vi "PromptForAttributes.vi"(9 "Attributes In":string[][](array[string]), 10 "Mouse Coords":T1, 11 "New Node Name":string) -> (2 "Canceled":bool, 3 "Attributes":string[][](array[string]))   [LabVIEW 2020]
uses:
  <vilib>/Utility/miscctls.llb/LVPoint32TypeDef.ctl
  Utils/FilePath.vi
  <vilib>/Utility/Data Type/NI_Data Type.lvlib
panel:
  out "Array":variant[](array[variant])
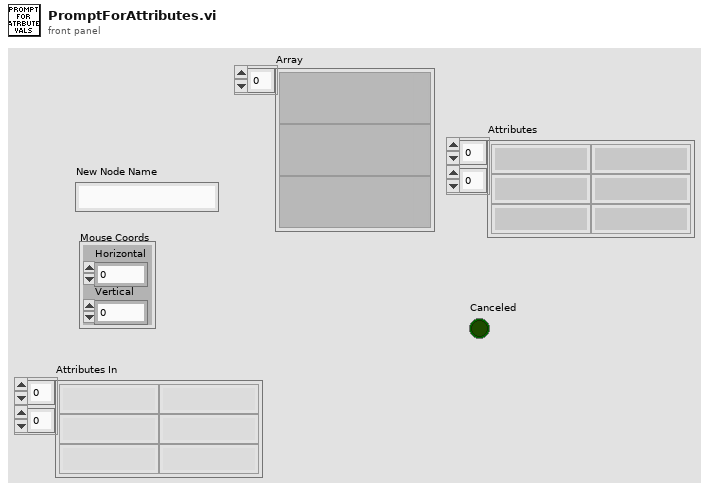
[diagram p1: front panel]
types:
  T1 = typedef "LVPoint32TypeDef.ctl" = cluster{"Horizontal":i32, "Vertical":i32}
  T2 = cluster{"Horizontal":i32, "Vertical":i32, "Horizontal":i32, "Vertical":i32}
  T3 = typedef "NI_Data Type.lvlib/Data Type.ctl" = enum8{"Invalid Type", "Void", "I8", "I16", "I32", "I64", "U8", "U16", "U32", "U64", "Single Float", "Double Float", "Extended Float", "Single Complex", "Double Complex", "Extended Complex", "Enum U8", "Enum U16", "Enum U32", "Enum U64", "Single Float With Unit", "Double Float With Unit", "Extended Float With Unit", "Single Complex with Unit", "Double Complex with Unit", "Extended Complex with Unit", "Boolean", "String", "Path", "Picture", "Tag", "Array", "Cluster", "Variant", "LV Variant", "Waveform", "Timestamp", "Digital Waveform", "Digital Data", "ExpressData", "Refnum", "External Data", "VI", "Poly VI", "LabVIEW Class Instance", "Fixed Point", "Set Collection", "Map Collection"}
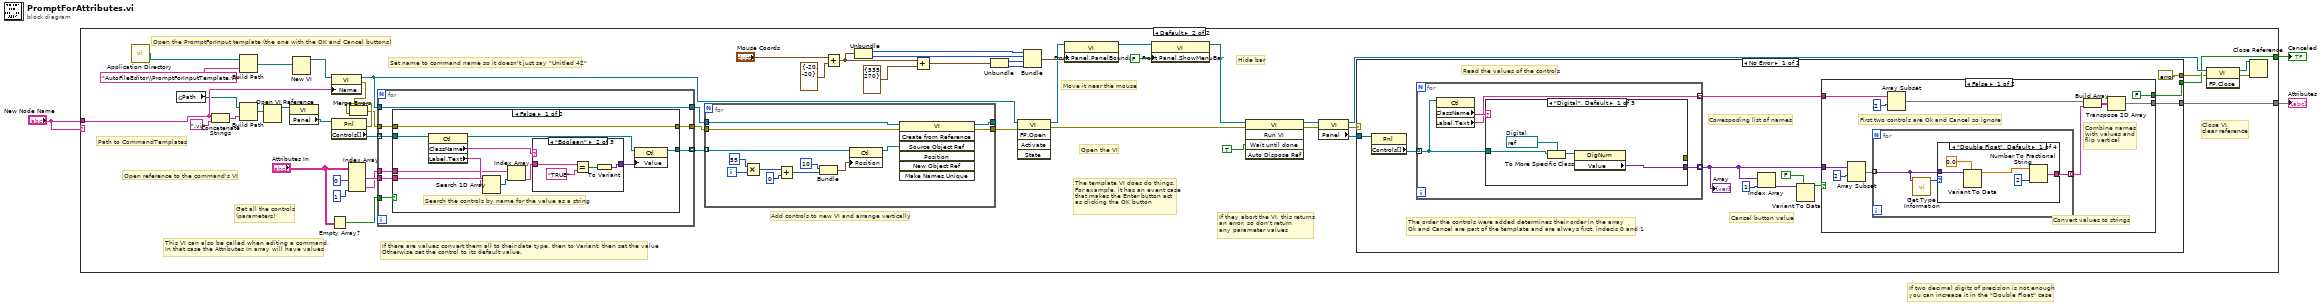
[diagram p0: block diagram]
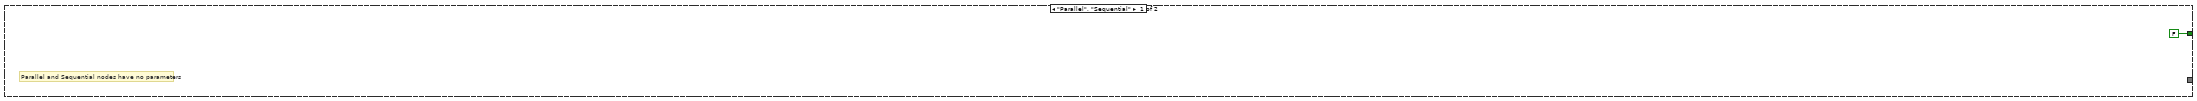
[diagram p2: hidden frame]
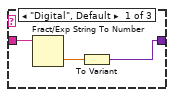
[diagram p3: hidden frame]
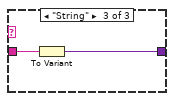
[diagram p4: hidden frame]
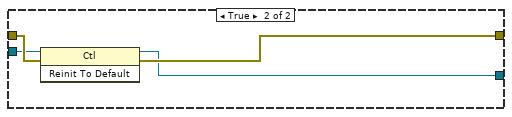
[diagram p5: hidden frame]
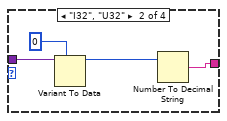
[diagram p6: hidden frame]
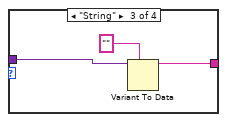
[diagram p7: hidden frame]
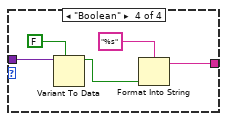
[diagram p8: hidden frame]
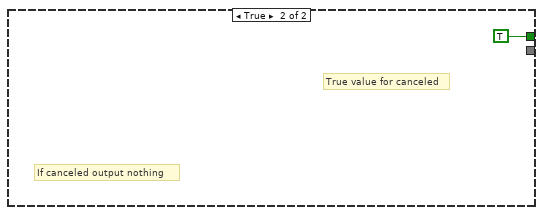
[diagram p9: hidden frame]
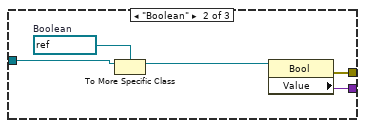
[diagram p10: hidden frame]
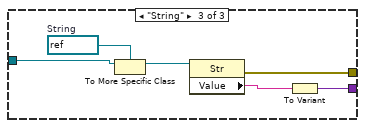
[diagram p11: hidden frame]
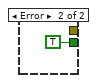
[diagram p12: hidden frame]
diagram:
  # "If two decimal digits of precision is not enough\nyou can increase it in the \"Double Float\" case"
  n1 = case shown="Default" "New Node Name" {
    tunnel: "New Node Name" -> [_ w13]
    tunnel: [FALSE ("Canceled") w42] -> w3
    tunnel: [_ w41] -> w2
    frame "Parallel", "Sequential" {
      # "Parallel and Sequential nodes have no parameters"
    }
    frame Default {
      # "The template VI does do things.\nFor example, it has an event case\nthat makes the Enter button act\nas clicking the OK button"
      # "Hide bar"
      # "Close VI,\nclear reference"
      # "If there are values convert them all to their data type, then to Variant, then set the value\nOtherwise set the control to its default value."
      # "This VI can also be called when editing a command.\nIn that case the Attributes In array will have values"
      # "Set name to command name so it doesn't just say \"Unitled 42\""
      # "Open the VI"
      # "Get all the controls\n(parameters)"
      # "Path to CommandTemplates"
      # "If they abort the VI, this returns\nan error, so don't return\nany parameter values"
      # "Open reference to the command's VI"
      # "Move it near the mouse"
      # "Add controls to new VI and arrange vertically"
      # "Open the PromptForInput template (the one with the OK and Cancel buttons)"
      n2 = call <vilib>:"Application Directory.vi"() -> ("Application Directory"=w11:path)
      n3 = global read "FilePath.vi" "Path"() -> (w12:path)
      n4 = Concatenate Strings(w13, ".vi" ("string")) -> (w45:string)
      n5 = Build Path(base path=w11, name or relative path="AutoFileEditor\\PromptForInputTemplate.vi") -> (appended path=w47:path)
      n6 = Build Path(base path=w12, name or relative path=w45) -> (appended path=w44:path)
      n7 = Open VI Reference(vi path=w44) -> (vi reference=w26:refnum<vi>)  [unwired: 5 in, 1 out]
      n8 = property class="VI"(reference=w26) -> ("Panel"=w56:refnum<vi>)  [unwired: 1 in, 2 out]
      n9 = New VI(10:w47) -> (3:w51:refnum<vi>)  [unwired: 6 in, 1 out]
      n10 = Empty Array?(array="Attributes In") -> (empty?=w14:bool)
      n11 = property class="Pnl"(reference=w56) -> (error out=w9:errorcluster, "Controls[]"=w22:refnum<vi>[])  [unwired: 1 in, 1 out]
      n12 = property class="VI"(reference=w51, "Name"=w13) -> (reference out=w5:refnum<vi>, error out=w8:errorcluster)  [unwired: 1 in]
      n13 = Index Array(array="Attributes In", index (col) #1=0 ("disabled index (col)"), index (col) #2=1 ("index (col)")) -> (element #1=w18:string[], element #2=w16:string[])  [unwired: 2 in]
      n14 = Merge Errors(w8, w9) -> (w7:errorcluster)
      n15 = for {
        tunnel: w22 -> [w62] mode=indexing
        tunnel: [w63] -> w21 mode=indexing
        tunnel: [w57] -> w20
        tunnel: w7 -> [w58]
        tunnel: [w64] -> w6
        tunnel: w5 -> [w64]
        tunnel: w18 -> [w61]
        tunnel: w16 -> [w60]
        tunnel: w14 -> [w59]
        n16 = case shown="False" w59 {
          tunnel: [w66 w86] -> w63
          tunnel: w62 -> [w75 w85]
          tunnel: w61 -> [w73 _]
          tunnel: w60 -> [w71 _]
          tunnel: w58 -> [w67 w88]
          tunnel: [w67 w87] -> w57
          frame False {
            # "Search the controls by name for the value as a string"
            n17 = property class="Ctl"(reference=w75) -> (reference out=w65:refnum<vi>, "ClassName"=w74:string, "Label.Text"=w72:string)  [unwired: 1 in, 1 out]
            n18 = Search 1D Array(1D array=w73, element=w72) -> (index of element=w70:i32)  [unwired: 1 in]
            n19 = Index Array(array=w71, index=w70) -> (element=w69:string)
            n20 = case shown="\"Boolean\"" w74 {
              tunnel: w69 -> [w78 w82 w84]
              tunnel: [w76 w79 w83] -> w68
              frame "Digital", Default {
                n21 = Fract/Exp String To Number(string=w78) -> (number=w77:dbl)  [unwired: 3 in, 1 out]
                n22 = To Variant(anything=w77) -> (Variant=w76:variant)
              }
              frame "Boolean" {
                n23 = Equal?(x=w82, y="TRUE") -> (x = y?=w80:bool)
                n24 = To Variant(anything=w80) -> (Variant=w79:variant)
              }
              frame "String" {
                n25 = To Variant(anything=w84) -> (Variant=w83:variant)
              }
            }
            n26 = property class="Ctl"(reference=w65, "Value"=w68) -> (reference out=w66:refnum<vi>)  [unwired: 1 in, 1 out]
          }
          frame True {
            n27 = invoke class="Ctl" method="Reinit To Default"(reference=w85, error in=w88) -> (reference out=w86:refnum<vi>, error out=w87:errorcluster)  [unwired: 1 in, 1 out]
          }
        }
      }
      n28 = for {
        tunnel: w6 -> [w163]
        tunnel: w20 -> [w162]
        tunnel: w21 -> [w151] mode=indexing
        tunnel: [w161] -> _
        tunnel: [w160] -> w10
        i -> [w159]
        n29 = Multiply(x=55, y=w159) -> (x*y=w157:i32)
        n30 = Add(x=w157, y=0) -> (x+y=w154:i32)
        n31 = Bundle("y"=10, w154) -> (w152:cluster{"y":i32, i32})  [unwired: 1 in]
        n32 = property class="Ctl"(reference=w151, "Position"=w152) -> (reference out=w155:refnum<vi>)  [unwired: 1 in, 1 out]
        n33 = invoke class="VI" method="Create from Reference"(reference=w163, error in=w162, "Source Object Ref"=w155) -> (reference out=w161:refnum<vi>, error out=w160:errorcluster)  [unwired: 4 in, 5 out]
      }
      n34 = Add(x="Mouse Coords", y=T1 {"Horizontal"=-20, "Vertical"=-20}) -> (x+y=w28:T1)
      n35 = Unbundle(w28) -> ("Horizontal"=w35:i32, "Vertical"=w34:i32)
      n36 = Add(x=w28, y=cluster{"Left":i16, "Top":i16} {"Left"=535, "Top"=270} ("Front Panel Window:Panel Bounds")) -> (x+y=w37:T1)
      n37 = Unbundle(w37) -> ("Horizontal"=w33:i32, "Vertical"=w32:i32)
      n38 = invoke class="VI" method="FP.Open"(reference=w5, error in=w10) -> (reference out=w25:refnum<vi>, error out=w50:errorcluster)  [unwired: 3 in, 3 out]
      n39 = Bundle("Horizontal"=w35, "Vertical"=w34, "Horizontal"=w33, "Vertical"=w32) -> (w31:T2)  [unwired: 1 in]
      n40 = property class="VI"(reference=w25, "Front Panel.PanelBounds"=w31) -> (reference out=w24:refnum<vi>)  [unwired: 1 in, 1 out]
      n41 = property class="VI"(reference=w24, "Front Panel.ShowMenuBar"=FALSE ("Front Panel Window:Show Menu Bar")) -> (reference out=w23:refnum<vi>)  [unwired: 1 in, 1 out]
      n42 = invoke class="VI" method="Run VI"(reference=w23, error in=w50, "Wait until done"=TRUE ("Wait Until Done")) -> (reference out=w52:refnum<vi>, error out=w53:errorcluster)  [unwired: 2 in, 3 out]
      n43 = property class="VI"(reference=w52, error in=w53) -> (reference out=w55:refnum<vi>, error out=w43:errorcluster, "Panel"=w54:refnum<vi>)
      n44 = case shown="No Error" w43 {
        tunnel: w54 -> [w98 _]
        tunnel: [w94 TRUE ("Canceled")] -> w42
        tunnel: [w91 _] -> w41
        tunnel: [errorcluster {"status"=FALSE, "code"=0, "source"=""} ("error constant") _] -> w38
        frame No Error {
          # "The order the controls were added determines their order in the array\nOk and Cancel are part of the template and are always first, indecis 0 and 1"
          # "Correspoding list of names"
          # "Cancel button value"
          # "Read the values of the controls"
          n45 = property class="Pnl"(reference=w98) -> ("Controls[]"=w99:refnum<vi>[])  [unwired: 1 in, 2 out]
          n46 = for {
            tunnel: w99 -> [w134] mode=indexing
            tunnel: [w132] -> w93 mode=indexing
            tunnel: [w131] -> w90 mode=indexing
            n47 = property class="Ctl"(reference=w134) -> ("ClassName"=w133:string, "Label.Text"=w131:string)  [unwired: 1 in, 2 out]
            n48 = case shown="\"Digital\", Default" w133 {
              tunnel: [_ w141 w147] -> _
              tunnel: w134 -> [w136 w140 w146]
              tunnel: [w135 w139 w144] -> w132
              frame "Digital", Default {
                w138 = refnum<vi> refnum  # Digital
                n49 = To More Specific Class(target class=w138, reference=w136) -> (specific class reference=w137:refnum<vi>)  [unwired: 1 in, 1 out]
                n50 = property class="DigNum"(reference=w137) -> ("Value"=w135:variant)  [unwired: 1 in, 2 out]
              }
              frame "Boolean" {
                w143 = refnum<vi> refnum  # Boolean
                n51 = To More Specific Class(target class=w143, reference=w140) -> (specific class reference=w142:refnum<vi>)  [unwired: 1 in, 1 out]
                n52 = property class="Bool"(reference=w142) -> (error out=w141:errorcluster, "Value"=w139:variant)  [unwired: 1 in, 1 out]
              }
              frame "String" {
                w149 = refnum<vi> refnum  # String
                n53 = To More Specific Class(target class=w149, reference=w146) -> (specific class reference=w148:refnum<vi>)  [unwired: 1 in, 1 out]
                n54 = property class="Str"(reference=w148) -> (error out=w147:errorcluster, "Value"=w145:string)  [unwired: 1 in, 1 out]
                n55 = To Variant(anything=w145) -> (Variant=w144:variant)
              }
            }
          }
          "Array" <- w93
          n56 = Index Array(array=w93, index=1) -> (element=w97:variant)
          n57 = Variant To Data(type=FALSE, Variant=w97) -> (data=w95:bool)  [unwired: 1 in, 1 out]
          n58 = case shown="False" w95 {
            tunnel: [FALSE ("Wait Until Done") TRUE ("Wait Until Done")] -> w94
            tunnel: w93 -> [w108 _]
            tunnel: [w100 _] -> w91
            tunnel: w90 -> [w103 _]
            frame False {
              # "Combine names\nwith values and\nflip vertical"
              # "First two controls are Ok and Cancel so ignore"
              # "Convert values to strings"
              n59 = Array Subset(array=w108, index=2) -> (w106:variant[])  [unwired: 1 in]
              n60 = for {
                tunnel: w106 -> [w111] mode=indexing
                tunnel: [w110] -> w105 mode=indexing
                n61 = call <vilib>:"Get Type Information.vi"("variant"=w111) -> ("type"=w112:T3)  [unwired: 6 in, 4 out]
                n62 = case shown="\"Double Float\", Default" w112 {
                  tunnel: w111 -> [w115 w120 w124 w129]
                  tunnel: [w113 w119 w122 w127] -> w110
                  frame "Double Float", Default {
                    n63 = Variant To Data(type=0.0, Variant=w115) -> (data=w117:dbl)  [unwired: 1 in, 1 out]
                    n64 = Number To Fractional String(number=w117, precision (6)=i16 2) -> (F-format string=w113:string)  [unwired: 2 in]
                  }
                  frame "I32", "U32" {
                    n65 = Variant To Data(type=i16 0 ("precision (6)"), Variant=w120) -> (data=w121:i16)  [unwired: 1 in, 1 out]
                    n66 = Number To Decimal String(number=w121) -> (decimal integer string=w119:string)  [unwired: 1 in]
                  }
                  frame "String" {
                    n67 = Variant To Data(type="", Variant=w124) -> (data=w122:string)  [unwired: 1 in, 1 out]
                  }
                  frame "Boolean" {
                    n68 = Variant To Data(type=FALSE ("Wait Until Done"), Variant=w129) -> (data=w125:bool)  [unwired: 1 in, 1 out]
                    n69 = Format Into String(format string="%s", w125) -> (resulting string=w127:string)  [unwired: 2 in, 1 out]
                  }
                }
              }
              n70 = Array Subset(array=w103, index=2) -> (w102:string[])  [unwired: 1 in]
              n71 = Build Array(w102, w105) -> (w101:string[][])
              n72 = Transpose 2D Array(2D array=w101) -> (transposed array=w100:string[][])
            }
            frame True {
              # "True value for canceled"
              # "If canceled output nothing"
            }
          }
        }
        frame Error {
        }
      }
      n73 = invoke class="VI" method="FP.Close"(reference=w55, error in=w38) -> (reference out=w40:refnum<vi>, error out=w39:errorcluster)  [unwired: 1 in, 1 out]
      n74 = Close Reference(reference=w40, error in (no error)=w39) -> ()  [unwired: 1 out]
    }
  }
  "Attributes" <- w2
  "Canceled" <- w3
